vi "ReadCSV.vi"(1 "Reinit":bool, 2 "File Path (.csv)":path=path "C:/Dropbox/Dr. Luke/AutoArchitectureTest/Demo Path 1.csv") -> (0 "Data (index by column)":dbl[][](array[numeric]))   [LabVIEW 2018]
uses:
  <vilib>/Utility/file.llb/Read Delimited Spreadsheet (DBL).vi
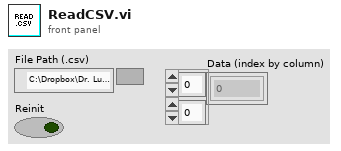
[diagram p1: front panel]
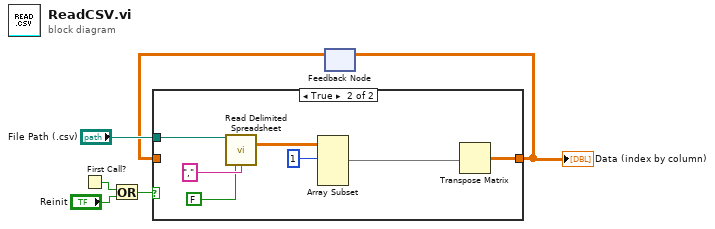
[diagram p0: block diagram]
diagram:
  n1 = First Call?() -> (First Call?: T/F=w2:bool)
  n2 = Or(x=w2, y="Reinit") -> (x .or. y?=w3:bool)
  n3 = feedback #1() -> (w4:dbl[][])  [unwired: 1 in]
  n4 = case shown="True" w3 {
    tunnel: "File Path (.csv)" -> [_ w14]
    tunnel: [w7 w9] -> w5
    tunnel: w4 -> [w7 _]
    frame False {
    }
    frame True {
      n5 = call-poly <vilib>:"Read Delimited Spreadsheet.vi"("file path (dialog if empty)"=w14, "transpose? (F)"=FALSE, "delimiter (\\t)"="," ("delimiter (\\t)")) -> ("all rows"=w11:dbl[][])  [unwired: 7 in, 5 out]
      n6 = Array Subset(array=w11, index (row)=1 ("index")) -> (w10:dbl[][])  [unwired: 3 in]
      n7 = Transpose Matrix(1:w10) -> (0:w9:dbl[][])
    }
  }
  "Data (index by column)" <- w5
  n8 = feedback-in #1(w5) -> ()
